vi "Sycronous Clock Frequency.vi"(10 "Clock":dbl, 11 "Frequency in":dbl) -> (2 "Points per sine wave":i32, 3 "Frequency out":dbl)   [LabVIEW 2021]
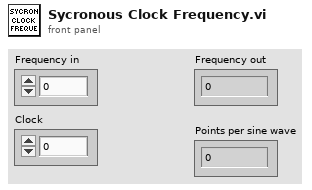
[diagram p1: front panel]
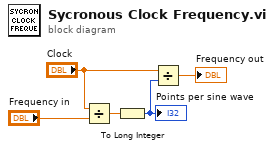
[diagram p0: block diagram]
diagram:
  n1 = Divide(x="Clock", y="Frequency in") -> (x/y=w4:dbl)
  n2 = To Long Integer(number=w4) -> (32bit integer=w2:i32)
  "Points per sine wave" <- w2
  n3 = Divide(x="Clock", y=w2) -> (x/y=→"Frequency out":dbl)
